vi "Get Library.vi"(8 "error in":errorcluster, 10 "library name":string, 11 "project ref":refnum<vi>) -> (0 "error out":errorcluster, 1 "found":bool, 2 "library item":refnum<vi>, 3 "project ref out":refnum<vi>)   [LabVIEW 2021, in "InstrumentStudio Plug-In Editor.lvlib"]
uses:
  InstrumentStudio Plug-In Editor.lvlib
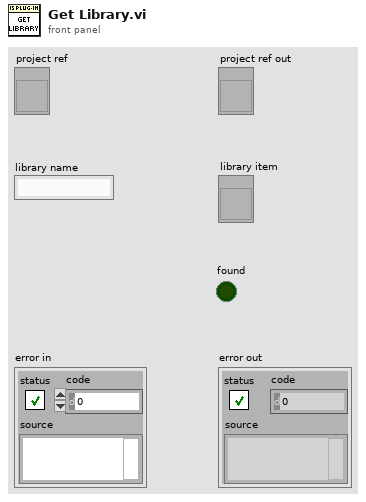
[diagram p1: front panel]
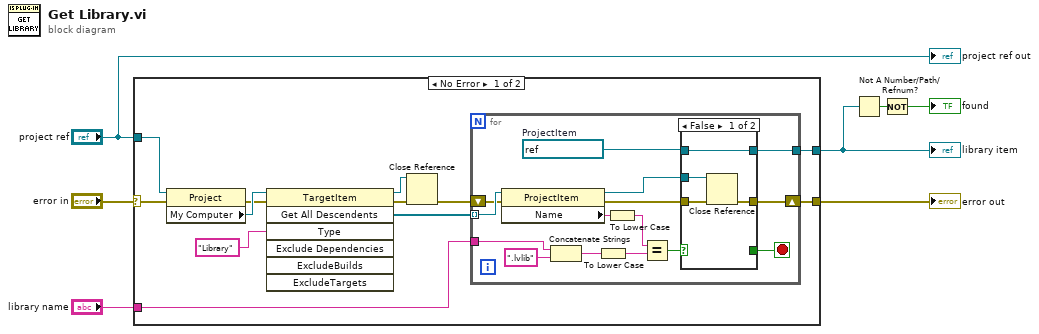
[diagram p0: block diagram]
diagram:
  n1 = case shown="No Error" "error in" {
    selector: "error in" -> [w15 w42]
    tunnel: "project ref" -> [w19 _]
    tunnel: "library name" -> [w9 _]
    tunnel: [w14 w42] -> w3
    tunnel: [w10 _] -> w4
    frame No Error {
      n2 = property class="Project"(reference=w19, error in=w15) -> (error out=w17:errorcluster, "My Computer"=w18:refnum<vi>)  [unwired: 1 out]
      n3 = invoke class="TargetItem" method="Get All Descendents"(reference=w18, error in=w17, "Type"="Library") -> (reference out=w12:refnum<vi>, error out=w13:errorcluster, "All Descendents"=w16:refnum<vi>[])  [unwired: 4 in, 4 out]
      n4 = Close Reference(reference=w12, error in (no error)=w13) -> (error out=w11:errorcluster)
      n5 = for {
        tunnel: w16 -> [w34] mode=indexing
        tunnel: w9 -> [w33]
        shift-right: [w27] -> w14
        shift-left: w11 -> [w31]
        tunnel: [w26] -> w10
        stop <- w21 stop-if-true
        w20 = refnum<vi> refnum  # ProjectItem
        n6 = property class="ProjectItem"(reference=w34, error in=w31) -> (reference out=w29:refnum<vi>, error out=w30:errorcluster, "Name"=w23:string)
        n7 = Concatenate Strings(w33, ".lvlib" ("string")) -> (w25:string)
        n8 = To Lower Case(string=w25) -> (all lower case string=w24:string)
        n9 = To Lower Case(string=w23) -> (all lower case string=w22:string)
        n10 = Equal?(x=w22, y=w24) -> (x = y?=w28:bool)
        n11 = case shown="False" w28 {
          selector: w28 -> [_ w39]
          tunnel: w30 -> [w38 w41]
          tunnel: w29 -> [w35 w40]
          tunnel: [w37 w41] -> w27
          tunnel: [w36 w40] -> w26
          tunnel: w20 -> [w36 _]
          tunnel: [_ w39] -> w21
          frame False {
            n12 = Close Reference(reference=w35, error in (no error)=w38) -> (error out=w37:errorcluster)
          }
          frame True {
          }
        }
      }
    }
    frame Error {
    }
  }
  "error out" <- w3
  "library item" <- w4
  n13 = Not A Number/Path/Refnum?(number/path/refnum=w4) -> (NaN/Path/Refnum?=w2:bool)
  n14 = Not(x=w2) -> (.not. x?=→"found":bool)
  "project ref out" <- "project ref"
